vi "Get Generic Export Signal.vi"(0 "Signal In":T1, 11 "error in":errorcluster) -> (4 "Generic Signal Out":i32(ring)=12487 items=["AI Convert Clock"=12484, "10MHz Reference Clock"=12536, "20MHz Timebase Clock"=12486, "Sample Clock"=12487, "Advance Trigger"=12488, "Reference Trigger"=12490, "Start Trigger"=12491, "Advance Complete Event"=12492, "AI Hold Complete Event"=12493, "Counter Output Event"=12494, "Change Detection Event"=12511, "Watchdog Timer Expired Event"=12512], 15 "error out":errorcluster)   [LabVIEW 2021, in "DAQ_Synchronization.lvlib"]
doc: "<B>Get Generic Export Signal</B> VI converts the input <B>signal</B> which are specific to TestScale and cDAQ devices into <B>generic export signals</B> with its equivalent enum values as supported by DAQmx Export signal VI."
uses:
  DAQ_Synchronization.lvlib
  Typedefs/Routing Signal.ctl
panel:
  # "Inputs"
  # "Outputs"
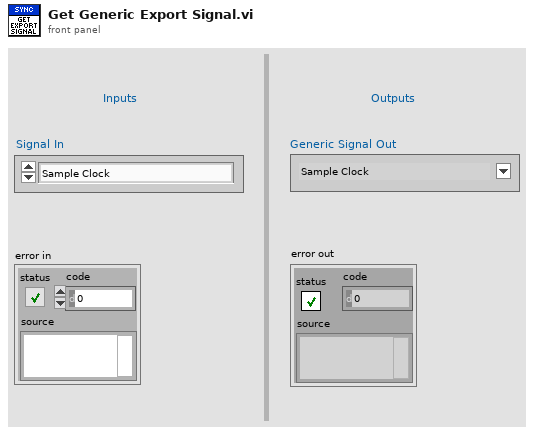
[diagram p1: front panel]
types:
  T1 = typedef "DAQ_Synchronization.lvlib/Routing Signal.ctl" = enum16{"Sample Clock", "Start Trigger"}
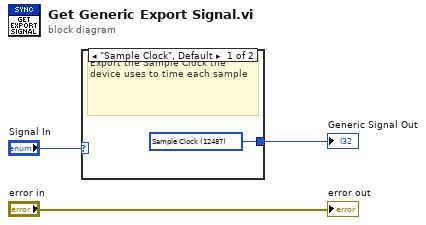
[diagram p0: block diagram]
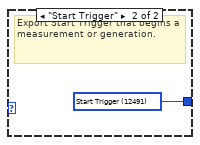
[diagram p2: hidden frame]
diagram:
  n1 = case shown="\"Sample Clock\", Default" "Signal In" {
    tunnel: [w4 w5] -> w1
    frame "Sample Clock", Default {
      w4 = 12487 items=["AI Convert Clock"=12484, "10MHz Reference Clock"=12536, "20MHz Timebase Clock"=12486, "Sample Clock"=12487, "Advance Trigger"=12488, "Reference Trigger"=12490, "Start Trigger"=12491, "Advance Complete Event"=12492, "AI Hold Complete Event"=12493, "Counter Output Event"=12494, "Change Detection Event"=12511, "Watchdog Timer Expired Event"=12512] ("signal")
      # "Export the Sample Clock the device uses to time each sample"
    }
    frame "Start Trigger" {
      w5 = 12491 items=["AI Convert Clock"=12484, "10MHz Reference Clock"=12536, "20MHz Timebase Clock"=12486, "Sample Clock"=12487, "Advance Trigger"=12488, "Reference Trigger"=12490, "Start Trigger"=12491, "Advance Complete Event"=12492, "AI Hold Complete Event"=12493, "Counter Output Event"=12494, "Change Detection Event"=12511, "Watchdog Timer Expired Event"=12512] ("signal")
      # "Export Start Trigger that begins a measurement or generation."
    }
  }
  "Generic Signal Out" <- w1
  "error out" <- "error in"
